vi "2D_array_interpolation_check (子VI).vi"(6 "yi":dbl, 9 "xi":dbl, 10 "x信号个数":i32, 11 "y信号个数":i32) -> (3 "布尔":bool)   [LabVIEW 2013]
doc: "本VI是2D矩阵插值VI中的一部分，用于判断输入值是否有误，如有误则报错，使得后续的插值操作不进行。"
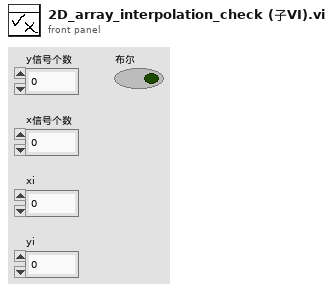
[diagram p1: front panel]
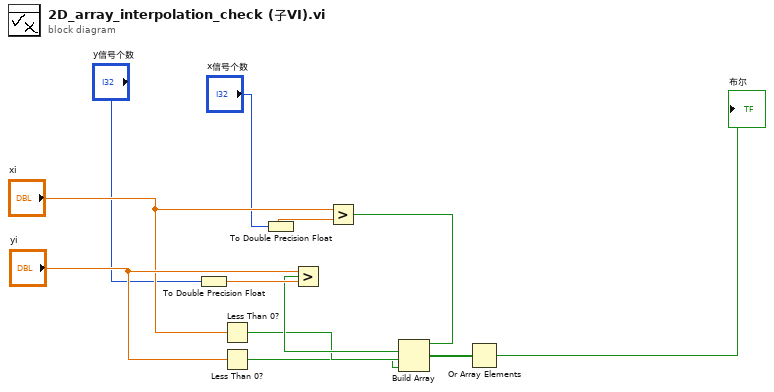
[diagram p0: block diagram]
diagram:
  n1 = To Double Precision Float(number="y信号个数") -> (double precision float=w9:dbl)
  n2 = Less Than 0?(x="xi") -> (x < 0?=w5:bool)
  n3 = Less Than 0?(x="yi") -> (x < 0?=w4:bool)
  n4 = To Double Precision Float(number="x信号个数") -> (double precision float=w8:dbl)
  n5 = Greater?(x="yi", y=w9) -> (0:w6:bool)
  n6 = Greater?(x="xi", y=w8) -> (0:w7:bool)
  n7 = Build Array(w7, w6, w5, w4) -> (w3:bool[])
  n8 = Or Array Elements(Boolean array=w3) -> (logical OR=→"布尔":bool)
